vi "3-lorentzian-heat-response -- analytic derivatives -- grad and curvature -- V4 -- test.vi"(10 "ω (rad/sec)":dbl=5.523060609045438 format="%#_10f") -> (0 "second derivatives map out":map{i32[], cdb}(c390), 1 "grad map  out":map{i32, cdb}(c390), 2 "ω out (rad/sec)":dbl=0.1 format="%#_10f", 3 "R(ω)":cdb=0.1+0.0i format="%#_10f")   [LabVIEW 2020]
uses:
  3-lorentzian-parameters.ctl
  3-lorentzian-heat-response action.ctl
panel:
  out "string IN":string="uuunumbersfunc[ 0.100000000000000006000000, {  ζ ->  0.688170999999999866000000,  τ1 ->  1.141804000000000040000000,  τS ->  0.521527999999999880000000 ,  τN ->  0.521527999999999880000000 ,  τC ->  3.436231999999999950000000 ,  κ0  ->  0.149712386031999989000000 } ] -  \r\r{  {  -0.013444022088146127500000    -0.036738300842769577900000  I     ,  0.004232653484324629300000    -0.000688064093116829735000  I     ,  -0.014412857413983033000000    -0.035210463626171965800000  I     ,  -0.010258767363036120500000    -0.036381813787190374300000  I     ,  0.024706242747499353900000    -0.001776881250200525780000  I     ,  0.018649656597092081200000  +     0.035268370018011981100000  I          }   ,  \r {  0.004232653484324629300000    -0.000688064093116829735000  I     ,  -0.004683245961566845190000    -0.030738701160948532500000  I     ,  0.005045561557296314620000    -0.000131206142178916458000  I     ,  -0.006511254259924059880000    -0.029021336117392434300000  I     ,  0.019619298462501058600000  +     0.000829603084398920950000  I     ,  0.011506670922022730800000  +     0.029460508647858610300000  I          }   ,  \r {  -0.014412857413983033000000    -0.035210463626171965800000  I     ,  0.005045561557296314620000    -0.000131206142178916458000  I     ,  -0.242865313621540096000000  +     0.115032549253587746000000  I     ,  -0.006194674208670073250000    -0.044058178001652369100000  I     ,  -0.032067598985382431100000    -0.171246267134601782000000  I     ,  0.231640059025370215000000    -0.158383416876224509000000  I          }   ,  \r {  -0.010258767363036120500000    -0.036381813787190374300000  I     ,  -0.006511254259924059880000    -0.029021336117392434300000  I     ,  -0.006194674208670073250000    -0.044058178001652369100000  I     ,  -0.247659655260382666000000  +     0.086047360373079570500000  I     ,  -0.012353576110863469200000    -0.172656803396370628000000  I     ,  0.246510542609008898000000    -0.130236744516910807000000  I          }   ,  \r {  0.024706242747499353900000    -0.001776881250200525780000  I     ,  0.019619298462501058600000  +     0.000829603084398920950000  I     ,  -0.032067598985382431100000    -0.171246267134601782000000  I     ,  -0.012353576110863469200000    -0.172656803396370628000000  I     ,  -1.754896628257085030000000  +     0.163828436513508202000000  I     ,  1.381383968000098990000000    -1.265280995624514570000000  I          }   ,  \r {  0.018649656597092081200000  +     0.035268370018011981100000  I     ,  0.011506670922022730800000  +     0.029460508647858610300000  I     ,  0.231640059025370215000000    -0.158383416876224509000000  I     ,  0.246510542609008898000000    -0.130236744516910807000000  I     ,  1.381383968000098990000000    -1.265280995624514570000000  I     ,  5.523060609045438160000000  +     2.430884904679364130000000  I          }      \r  }  \r"
  in  "κ0":dbl(slide)=0.284189643628 min=0.0 max=0.3 step=1e-12 scale=0.01..1.0 scale format="%#_3p"
  in  "ζ":dbl(slide)=2.189345 min=0.0 max=0.3 step=1e-06 scale=0.01..10.0 scale format="%#_3p"
  in  "τN":dbl(slide)=1.227454 min=0.0 max=0.3 step=1e-06 scale=0.01..10.0 scale format="%#_3p"
  in  "T1":dbl(slide)=0.17411599999999997 min=0.0 max=0.3 step=1e-06 scale=0.01..10.0 scale format="%#_3p"
  in  "τC":dbl(slide)=0.18537099999999995 min=0.0 max=0.3 step=1e-06 scale=0.01..10.0 scale format="%#_3p"
  in  "τS":dbl(slide)=1.639305 min=0.0 max=0.3 step=1e-06 scale=0.01..10.0 scale format="%#_3p"
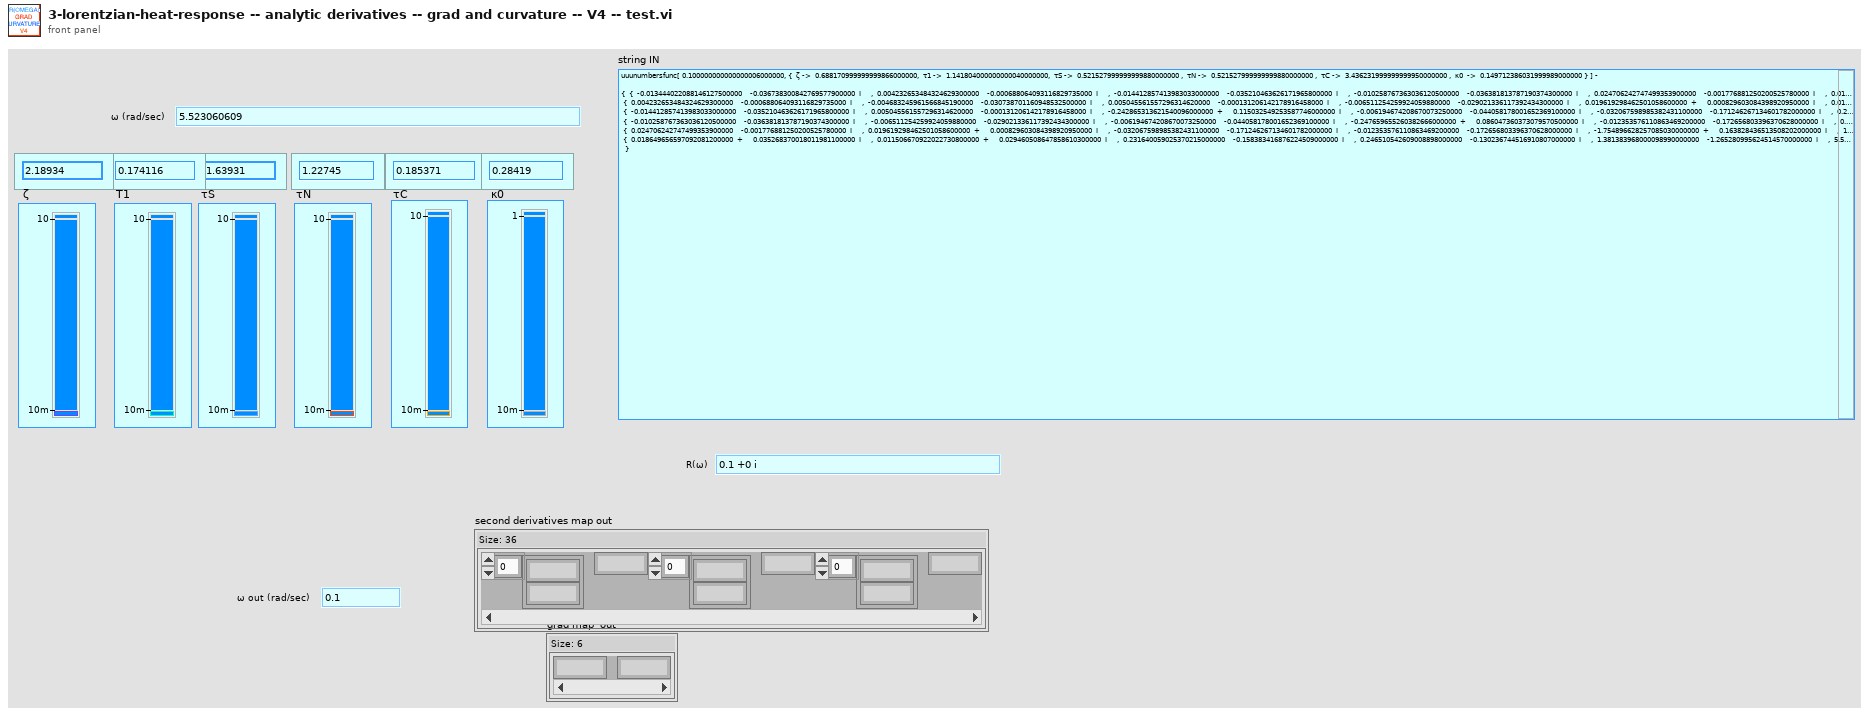
[diagram p1: front panel]
types:
  T1 = typedef "3-lorentzian-parameters.ctl" = enum16{"ζ", "τ1", "τS", "τN", "τC", "κ0", "m1", "m2", "m3", "T (K)", "B (T)", "θ (deg)"}
  T2 = typedef "3-lorentzian-heat-response action.ctl" = enum16{"calc R", "create string", "calc m1m2m3", "dζ", "dT1", "dτS", "dτN", "dτC", "d-all", "dκ0", "T(K)", "m1", "m2", "m3", "parse string", "θ (deg)", "B (T)"}
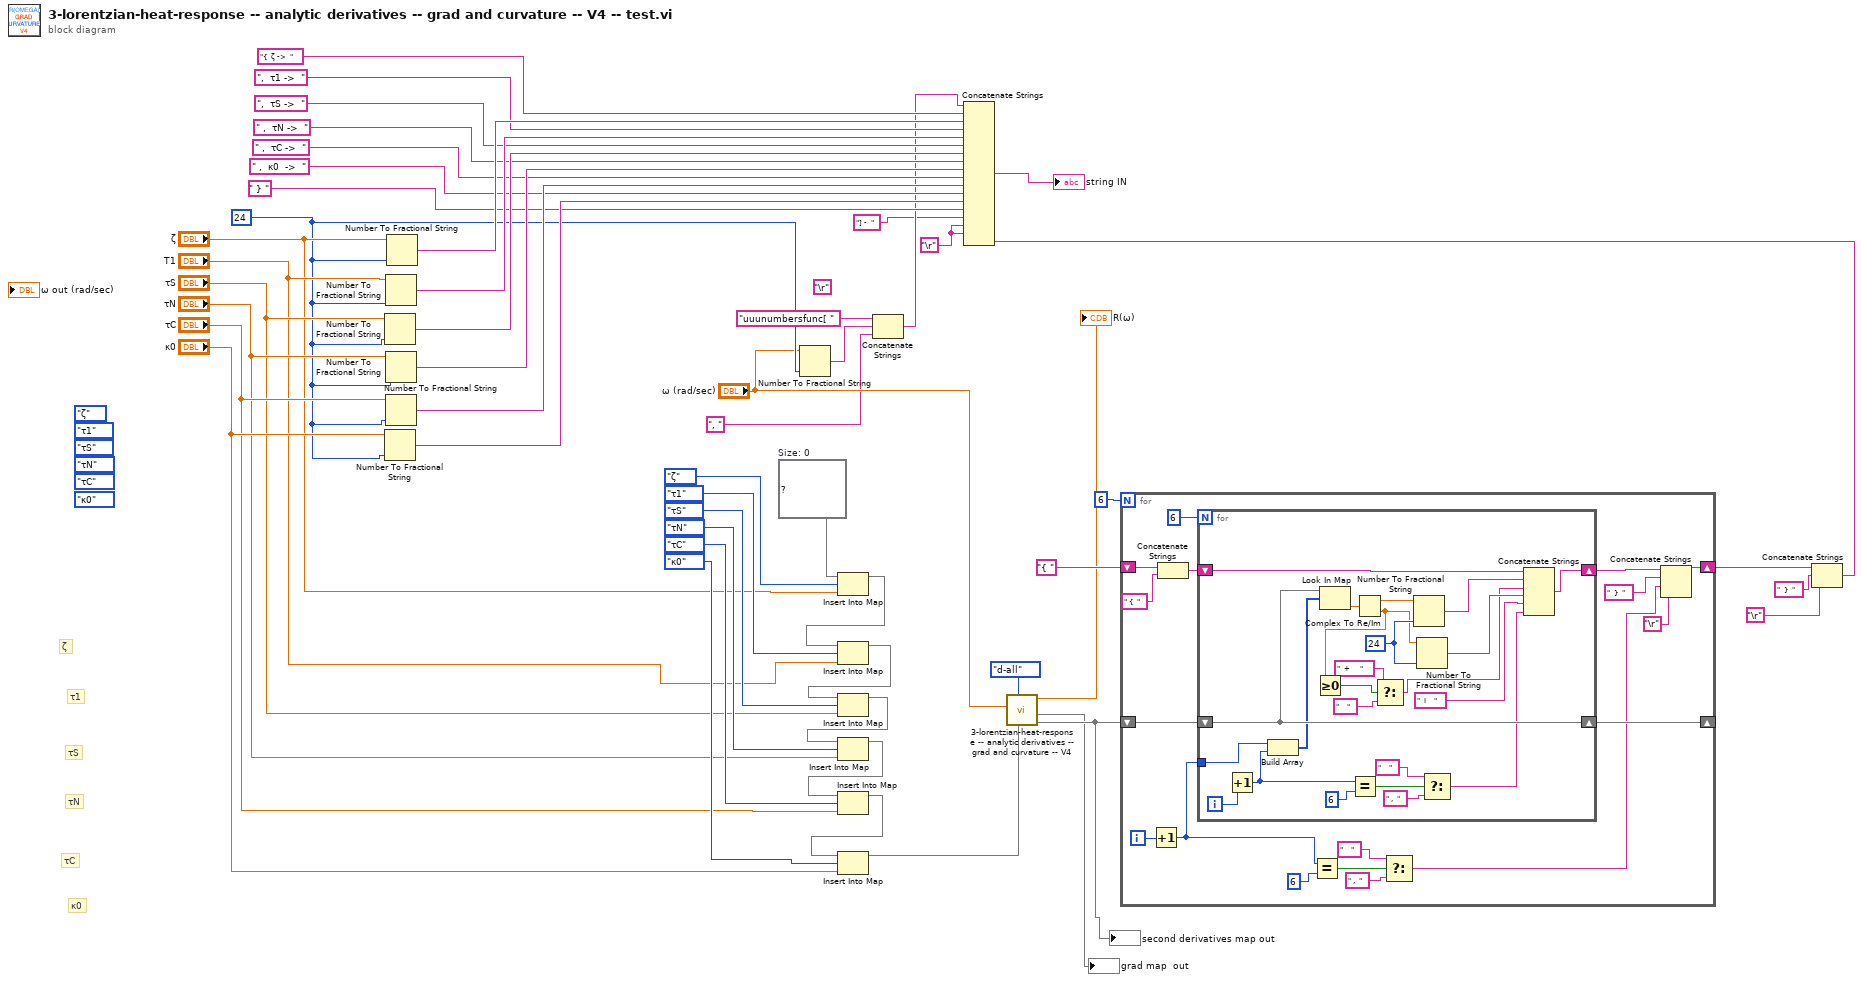
[diagram p0: block diagram]
diagram:
  (unwired) "\r"
  w35 = map{T1, dbl} {}  # Size: 0
  w37 = "\r"
  w16 = i16 24 ("precision (6)")
  (unwired) 3-lorentzian-parameters."κ0" ("Plost: sweep window")
  (unwired) 3-lorentzian-parameters."τC" ("Plost: sweep window")
  (unwired) 3-lorentzian-parameters."τN" ("Plost: sweep window")
  (unwired) 3-lorentzian-parameters."τS" ("Plost: sweep window")
  (unwired) 3-lorentzian-parameters."τ1" ("Plost: sweep window")
  (unwired) 3-lorentzian-parameters."ζ" ("Plost: sweep window")
  # "κ0"
  # "τC"
  # "τN"
  # "τS"
  # "τ1"
  # "ζ"
  n1 = Number To Fractional String(number="τS", precision (6)=w16) -> (F-format string=w45:string)  [unwired: 2 in]
  n2 = Number To Fractional String(number="κ0", precision (6)=w16) -> (F-format string=w39:string)  [unwired: 2 in]
  n3 = Number To Fractional String(number="T1", precision (6)=w16) -> (F-format string=w47:string)  [unwired: 2 in]
  n4 = Number To Fractional String(number="τN", precision (6)=w16) -> (F-format string=w43:string)  [unwired: 2 in]
  n5 = Number To Fractional String(number="τC", precision (6)=w16) -> (F-format string=w41:string)  [unwired: 2 in]
  n6 = Number To Fractional String(number="ζ", precision (6)=w16) -> (F-format string=w50:string)  [unwired: 2 in]
  n7 = Number To Fractional String(number="ω (rad/sec)", precision (6)=w16) -> (F-format string=w13:string)  [unwired: 2 in]
  n8 = Insert Into Map(map in=w35, key=3-lorentzian-parameters."ζ" ("Plost: sweep window"), value="ζ") -> (map out=w34:map{T1, dbl})  [unwired: 2 out]
  n9 = Insert Into Map(map in=w34, key=3-lorentzian-parameters."τ1" ("Plost: sweep window"), value="T1") -> (map out=w33:map{T1, dbl})  [unwired: 2 out]
  n10 = Insert Into Map(map in=w33, key=3-lorentzian-parameters."τS" ("Plost: sweep window"), value="τS") -> (map out=w32:map{T1, dbl})  [unwired: 2 out]
  n11 = Insert Into Map(map in=w32, key=3-lorentzian-parameters."τN" ("Plost: sweep window"), value="τN") -> (map out=w31:map{T1, dbl})  [unwired: 2 out]
  n12 = Insert Into Map(map in=w31, key=3-lorentzian-parameters."τC" ("Plost: sweep window"), value="τC") -> (map out=w30:map{T1, dbl})  [unwired: 2 out]
  n13 = Insert Into Map(map in=w30, key=3-lorentzian-parameters."κ0" ("Plost: sweep window"), value="κ0") -> (map out=w17:map{T1, dbl})  [unwired: 2 out]
  n14 = Concatenate Strings("uuunumbersfunc[ ", w13, ", ") -> (w12:string)
  n15 = call "3-lorentzian-heat-response -- analytic derivatives -- grad and curvature -- V4.vi"("parameters map  IN"=w17, "action"=3-lorentzian-heat-response_action."d-all", "ω (rad/sec)"="ω (rad/sec)") -> ("second derivatives map out"=w2:map{i32[], cdb}, "grad map  out"=→"grad map  out":map{i32, cdb}, "R(ω)"=→"R(ω)":cdb)  [unwired: 5 in, 1 out]
  "second derivatives map out" <- w2
  n16 = for {
    N: 6 -> [_]
    shift-right: [w65] -> _
    shift-left: w2 -> [w67]
    shift-right: [w61] -> w7
    shift-left: "{ " -> [w64]
    i -> [w66]
    n17 = Increment(x=w66) -> (x+1=w53:i32)
    n18 = Concatenate Strings(w64, " {  ") -> (w60:string)
    n19 = for {
      N: 6 -> [_]
      shift-right: [w89] -> w65
      shift-left: w67 -> [w89]
      tunnel: w53 -> [w90]
      shift-right: [w77] -> w59
      shift-left: w60 -> [w76]
      i -> [w91]
      w85 = i16 24 ("precision (6)")
      n20 = Increment(x=w91) -> (x+1=w84:i32)
      n21 = Build Array(w90, w84) -> (w88:i32[])
      n22 = Look In Map(map=w89, key=w88) -> (value=w87:cdb)  [unwired: 1 in, 1 out]
      n23 = Equal?(x=w84, y=6) -> (x = y?=w82:bool)
      n24 = Complex To Re/Im(x + iy=w87) -> (x=w86:dbl, y=w73:dbl)
      n25 = Greater Or Equal To 0?(x=w73) -> (x >= 0?=w72:bool)
      n26 = Select(t="  +     ", s=w72, f="    ") -> (s? t:f=w69:string)
      n27 = Number To Fractional String(number=w86, precision (6)=w85) -> (F-format string=w79:string)  [unwired: 2 in]
      n28 = Number To Fractional String(number=w73, precision (6)=w85) -> (F-format string=w78:string)  [unwired: 2 in]
      n29 = Select(t="    ", s=w82, f=" ,  ") -> (s? t:f=w75:string)
      n30 = Concatenate Strings(w76, w79, w69, w78, "  I    ", w75) -> (w77:string)
    }
    n31 = Equal?(x=w53, y=6) -> (x = y?=w56:bool)
    n32 = Select(t="    ", s=w56, f=" ,  ") -> (s? t:f=w52:string)
    n33 = Concatenate Strings(w59, "  }  ", w52, "\r") -> (w61:string)
  }
  n34 = Concatenate Strings(w7, "  }  ", "\r") -> (w6:string)
  n35 = Concatenate Strings(w12, "{  ζ ->  ", w50, ",  τ1 ->  ", w47, ",  τS ->  ", w45, " ,  τN ->  ", w43, " ,  τC ->  ", w41, " ,  κ0  ->  ", w39, " } ", "] -  ", w37, w37, w6) -> (→"string IN":string)
